vi "Optimal Offset Calculations.vi"(4 "Decay Normalization Factor":dbl, 6 "Weighted Fit":bool, 8 "Error In":errorcluster, 9 "Polynomial":enum16{"pol2", "pol4"}(ring)=enum."pol4", 10 "Offset Array":dbl[](array[numeric]), 11 "Chi^2 Array":dbl[](array[numeric])) -> (0 "Error Out":errorcluster, 1 "C00":dbl, 2 "Chi^2":dbl, 3 "t0":dbl, 5 "Best Polynomial Fit":dbl[](array[numeric]), 7 "Offset Array used for Fit":dbl[](array[numeric]))   [LabVIEW 2021, in "Fits.lvlib"]
uses:
  Fits.lvlib
  <vilib>/gmath/zero.llb/Find All Zeros of f(x) (Formula).vi
  <vilib>/Analysis/NI_AALPro.lvlib
  Error/Error.lvlib
  <vilib>/gmath/NI_Gmath.lvlib
  Strings/Strings.lvlib
panel:
  out "Actual Minimum t0 Location":dbl
  out "Actual Minimum Chi^2":dbl
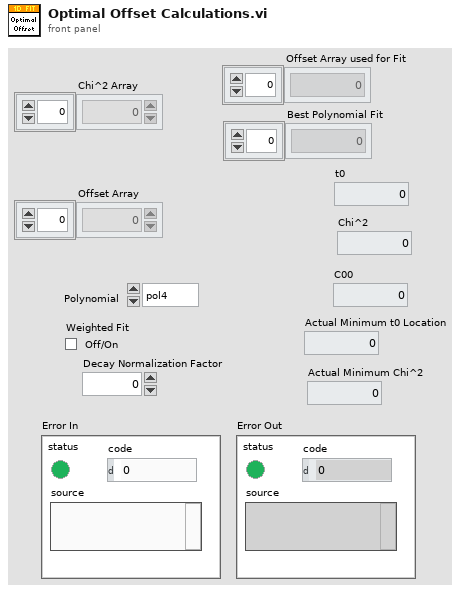
[diagram p1: front panel]
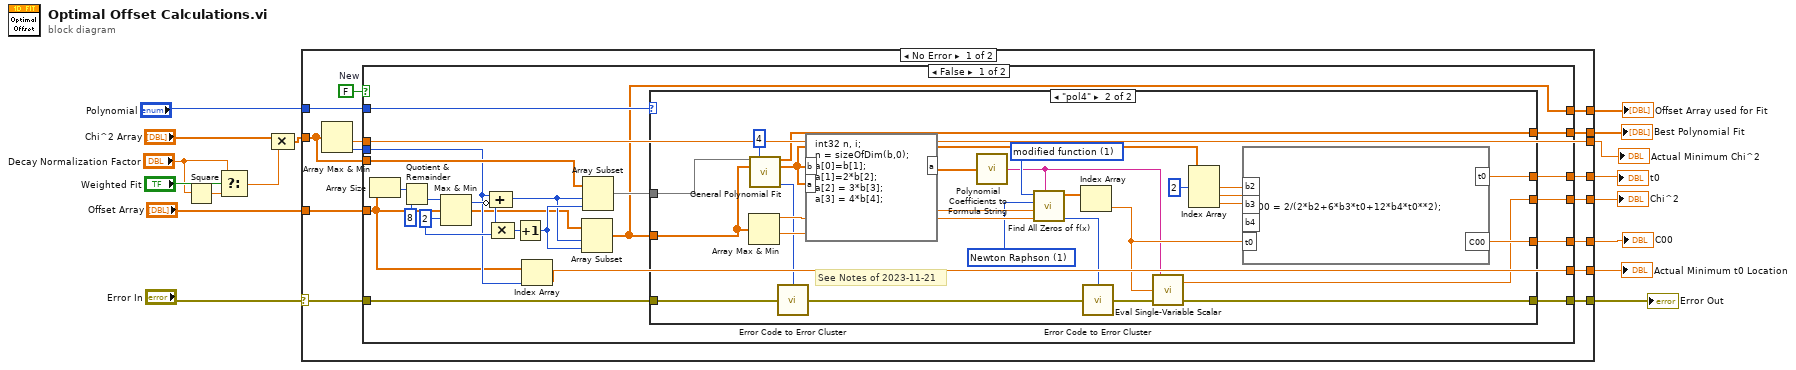
[diagram p0: block diagram]
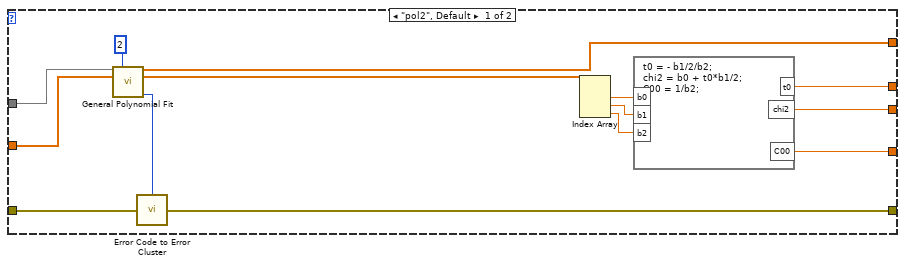
[diagram p2: hidden frame]
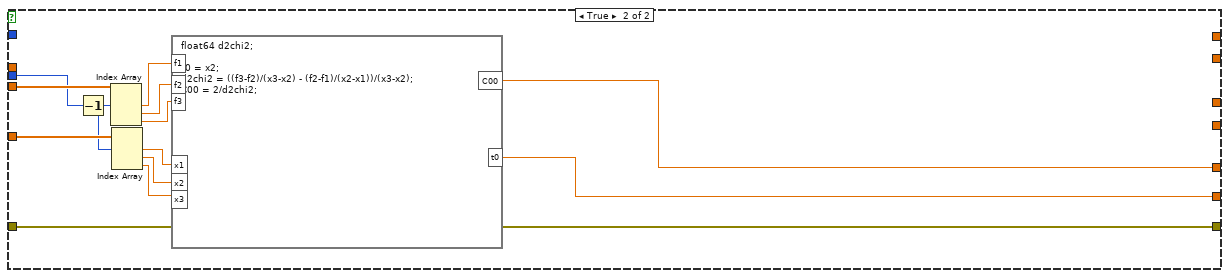
[diagram p3: hidden frame]
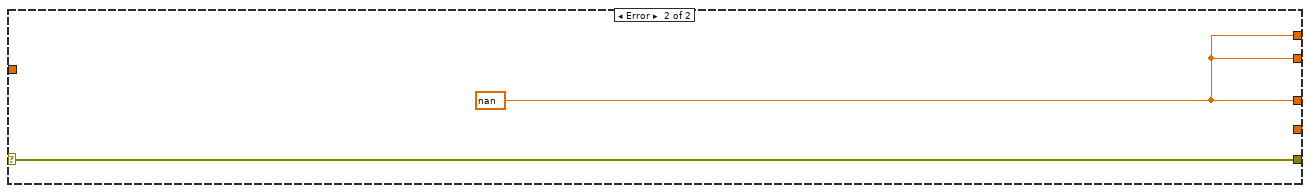
[diagram p4: hidden frame]
diagram:
  n1 = Square(x="Decay Normalization Factor") -> (x^2=w3:dbl)
  n2 = Select(t="Decay Normalization Factor", s="Weighted Fit", f=w3) -> (s? t:f=w1:dbl)
  n3 = Compound Arithmetic op=MULTIPLY("Chi^2 Array", w1) -> (w2:dbl[])
  n4 = case shown="No Error" "Error In" {
    selector: "Error In" -> [w26 w107]
    tunnel: "Offset Array" -> [w21 _]
    tunnel: [w31 w106] -> w16
    tunnel: [w30 w106] -> w15
    tunnel: [w29 w106] -> w14
    tunnel: [w28 _] -> w13
    tunnel: w2 -> [w24 _]
    tunnel: [w25 w107] -> w9
    tunnel: "Polynomial" -> [w27 _]
    tunnel: [w23 _] -> w8
    tunnel: [w18 _] -> w7
    tunnel: [w20 _] -> w6
    frame No Error {
      w19 = FALSE  # New
      n5 = Array Max & Min(array=w24) -> (min value=w18:dbl, min index (indices)=w22:i32)  [unwired: 2 out]
      n6 = case shown="False" w19 {
        tunnel: [w52 w95] -> w31
        tunnel: [w51 _] -> w30
        tunnel: [w50 _] -> w29
        tunnel: [w49 _] -> w28
        tunnel: w27 -> [w48 _]
        tunnel: w26 -> [w47 w93]
        tunnel: [w46 w93] -> w25
        tunnel: w24 -> [w45 w105]
        tunnel: [w35 _] -> w23
        tunnel: w22 -> [w34 w104]
        tunnel: w21 -> [w33 w103]
        tunnel: [w32 w94] -> w20
        tunnel: w18 -> [_ _]
        frame False {
          w40 = 2 ("y")
          n7 = Array Size(array=w33) -> (size(s)=w44:i32)
          n8 = Quotient & Remainder(x=w44, y=8) -> (floor(x/y)=w42:i32)  [unwired: 1 out]
          n9 = Max & Min(x=w42, y=w40) -> (max(x,y)=w41:i32)  [unwired: 1 out]
          n10 = Compound Arithmetic op=ADD(w34, invert w41) -> (w37:i32)
          n11 = Compound Arithmetic op=MULTIPLY(w41, w40) -> (w39:i32)
          n12 = Increment(x=w39) -> (x+1=w38:i32)
          n13 = Index Array(array=w33, index=w34) -> (element=w32:dbl)
          n14 = Array Subset(array=w33, index=w37, length=w38) -> (w35:dbl[])
          n15 = Array Subset(array=w45, index=w37, length=w38) -> (w36:dbl[])
          n16 = case shown="\"pol4\"" w48 {
            tunnel: [w66 w92] -> w52
            tunnel: [w65 w71] -> w51
            tunnel: [w64 w91] -> w50
            tunnel: [w59 w87] -> w49
            tunnel: w47 -> [w57 w78]
            tunnel: [w55 w73] -> w46
            tunnel: w36 -> [w54 w68]
            tunnel: w35 -> [w53 w67]
            frame "pol2", Default {
              n17 = call <vilib>:"General Polynomial Fit.vi"("Y"=w54, "polynomial order"=2, "X"=w53) -> ("Best Polynomial Fit"=w59:dbl[], "Polynomial Coefficients"=w60:dbl[], "error"=w56:i32)  [unwired: 9 in, 1 out]
              n18 = call "Error Code to Error Cluster.vi"("Error Code"=w56, "Error In"=w57) -> ("Error Out"=w55:errorcluster)  [unwired: 13 in]
              n19 = Index Array(array=w60) -> (element #1=w61:dbl, element #2=w62:dbl, element #3=w63:dbl)  [unwired: 3 in]
              n20 = formula code="t0 = - b1/2/b2;\nchi2 = b0 + t0*b1/2;\nC00 = 1/b2;"("b0"=w61, "b1"=w62, "b2"=w63) -> ("t0"=w64:dbl, "chi2"=w65:dbl, "C00"=w66:dbl)
            }
            frame "pol4" {
              w82 = u16 1 items=["fixed function", "modified function"] ("step type")
              w83 = u16 1 items=["Ridders", "Newton Raphson"] ("algorithm")
              # "See Notes of 2023-11-21"
              n21 = Array Max & Min(array=w67) -> (max value=w84:dbl, min value=w85:dbl)  [unwired: 2 out]
              n22 = call <vilib>:"General Polynomial Fit.vi"("Y"=w68, "polynomial order"=4, "X"=w67) -> ("Best Polynomial Fit"=w87:dbl[], "Polynomial Coefficients"=w70:dbl[], "error"=w77:i32)  [unwired: 9 in, 1 out]
              n23 = call "Error Code to Error Cluster.vi"("Error Code"=w77, "Error In"=w78) -> ("Error Out"=w75:errorcluster)  [unwired: 13 in]
              n24 = formula code="int32 n, i;\nn = sizeOfDim(b,0);\na[0]=b[1];\na[1]=2*b[2];\na[2] = 3*b[3];\na[3] = 4*b[4];"("b"=w70, "a"=w70) -> ("a"=w69:dbl[])
              n25 = call "Polynomial Coefficients to Formula String.vi"("Polynomial Coefficients"=w69) -> ("formula"=w72:string)  [unwired: 8 in]
              n26 = call-poly <vilib>:"Find All Zeros of f(x).vi"("formula"=w72, "end"=w84, "start"=w85, "algorithm"=w83, "step type"=w82) -> ("error"=w76:i32, "Zeros"=w81:dbl[])  [unwired: 3 in, 2 out]
              n27 = Index Array(array=w81) -> (element=w79:dbl)  [unwired: 1 in]
              n28 = call "Error Code to Error Cluster.vi"("Error Code"=w76, "Error In"=w75) -> ("Error Out"=w74:errorcluster)  [unwired: 13 in]
              n29 = call <vilib>:"Eval Single-Variable Scalar.vi"("error in (no error)"=w74, "x value"=w79, "formula"=w72) -> ("error out"=w73:errorcluster, "y value"=w71:dbl)
              n30 = Index Array(array=w70, index #1=2 ("index")) -> (element #1=w88:dbl, element #2=w89:dbl, element #3=w90:dbl)  [unwired: 2 in]
              n31 = formula code="C00 = 2/(2*b2+6*b3*t0+12*b4*t0**2);"("b2"=w88, "b3"=w89, "b4"=w90, "t0"=w79) -> ("t0"=w91:dbl, "C00"=w92:dbl)
            }
          }
        }
        frame True {
          n32 = Decrement(x=w104) -> (x-1=w102:i32)
          n33 = Index Array(array=w105, index #1=w102) -> (element #1=w101:dbl, element #2=w100:dbl, element #3=w99:dbl)  [unwired: 2 in]
          n34 = Index Array(array=w103, index #1=w102) -> (element #1=w98:dbl, element #2=w97:dbl, element #3=w96:dbl)  [unwired: 2 in]
          n35 = formula code="float64 d2chi2;\n\nt0 = x2;\nd2chi2 = ((f3-f2)/(x3-x2) - (f2-f1)/(x2-x1))/(x3-x2);\nC00 = 2/d2chi2;"("f3"=w99, "f2"=w100, "f1"=w101, "x1"=w98, "x2"=w97, "x3"=w96) -> ("C00"=w95:dbl, "t0"=w94:dbl)
        }
      }
    }
    frame Error {
      w106 = nan ("C00")
    }
  }
  "Chi^2" <- w15
  "C00" <- w16
  "t0" <- w14
  "Best Polynomial Fit" <- w13
  "Error Out" <- w9
  "Offset Array used for Fit" <- w8
  "Actual Minimum Chi^2" <- w7
  "Actual Minimum t0 Location" <- w6
